vi "Initialize.vi"(8 "error in (no error)":errorcluster, 9 "Reset (True)":bool=TRUE, 10 "ID Query (True)":bool=TRUE, 11 "VISA resource name":refnum<visa-resource-name>) -> (0 "error out":errorcluster, 3 "VISA resource name out":refnum<visa-resource-name>)   [LabVIEW 2010, in "Agilent U2722.lvlib"]
doc: "Establishes communication with the instrument and optionally performs an instrument identification query and/or an instrument reset. It also places the instrument in a default state needed for other instrument driver operations. Therefore, call this VI before calling other instrument driver VIs for this instrument. Generally, you need to call the Initialize VI only once at the beginning of an application."
uses:
  Agilent U2722.lvlib
panel:
  # "(c) 2009 National Instruments.  ALL RIGHTS RESERVED."
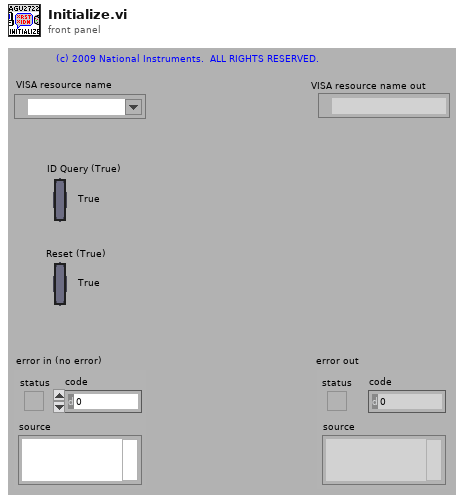
[diagram p1: front panel]
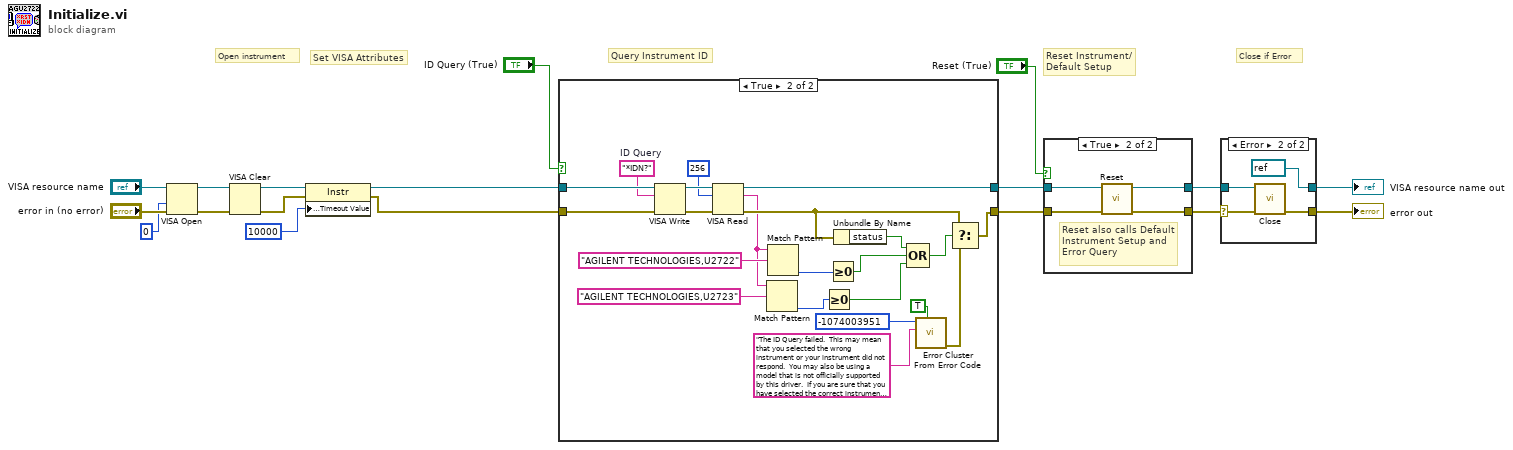
[diagram p0: block diagram]
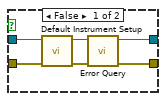
[diagram p3: hidden frame]
diagram:
  # "Set VISA Attributes"
  # "Close if Error"
  # "Query Instrument ID"
  # "Reset Instrument/\nDefault Setup"
  # "Open instrument"
  n1 = VISA Open(access mode=u32 0, error in (no error)="error in (no error)", VISA resource name="VISA resource name") -> (VISA resource name=w10:refnum<visa-resource-name>, error out=w9:errorcluster)  [unwired: 2 in]
  n2 = VISA Clear(VISA resource name=w10, error in (no error)=w9) -> (VISA resource name out=w8:refnum<visa-resource-name>, error out=w7:errorcluster)
  n3 = property class="Instr"(reference=w8, error in=w7, "General Settings:Timeout Value"=u32 10000) -> (reference out=w2:refnum<visa-resource-name>, error out=w1:errorcluster)
  n4 = case shown="True" "ID Query (True)" {
    tunnel: [w19 w42] -> w17
    tunnel: [w20 w39] -> w18
    tunnel: w2 -> [w20 w40]
    tunnel: w1 -> [w19 w41]
    frame False {
    }
    frame True {
      w34 = "*IDN?"  # ID Query
      n5 = VISA Write(VISA resource name=w40, write buffer=w34, error in (no error)=w41) -> (VISA resource name out=w38:refnum<visa-resource-name>, error out=w37:errorcluster)  [unwired: 1 out]
      n6 = VISA Read(VISA resource name=w38, byte count=u32 256, error in (no error)=w37) -> (VISA resource name out=w39:refnum<visa-resource-name>, read buffer=w23:string, error out=w28:errorcluster)  [unwired: 1 out]
      n7 = Match Pattern(string=w23, regular expression="AGILENT TECHNOLOGIES,U2723") -> (offset past match=w22:i32)  [unwired: 1 in, 3 out]
      n8 = Match Pattern(string=w23, regular expression="AGILENT TECHNOLOGIES,U2722") -> (offset past match=w29:i32)  [unwired: 1 in, 3 out]
      n9 = Greater Or Equal To 0?(x=w22) -> (x >= 0?=w21:bool)
      n10 = Greater Or Equal To 0?(x=w29) -> (x >= 0?=w26:bool)
      n11 = Unbundle By Name(w28) -> ("status"=w27:bool)
      n12 = Compound Arithmetic op=OR(w27, w26, w21) -> (w25:bool)
      n13 = call <vilib>:"Error Cluster From Error Code.vi"("show call chain? (False)"=TRUE, "error message (\"\")"="The ID Query failed.  This may mean that you selected the wrong instrument or your instrument did not respond.  You may also be using a model that is not officially supported by this driver.  If you are sure that you have selected the correct instrument and it is responding, try disabling the ID Query." ("Source (VI Name)"), "error code (0)"=-1074003951 ("Code")) -> ("error out"=w33:errorcluster)  [unwired: 6 in]
      n14 = Select(t=w28, s=w25, f=w33) -> (s? t:f=w42:errorcluster)
    }
  }
  n15 = case shown="True" "Reset (True)" {
    tunnel: w17 -> [w47 w49]
    tunnel: [w44 w52] -> w3
    tunnel: w18 -> [w48 w50]
    tunnel: [w45 w51] -> w4
    frame False {
      n16 = call "Default Instrument Setup.vi"("error in (no error)"=w47, "VISA resource name"=w48) -> ("error out"=w43:errorcluster, "VISA resource name out"=w46:refnum<visa-resource-name>)  [unwired: 8 in]
      n17 = call "Error Query.vi"("error in (no error)"=w43, "VISA resource name"=w46) -> ("error out"=w44:errorcluster, "VISA resource name out"=w45:refnum<visa-resource-name>)  [unwired: 6 in, 2 out]
    }
    frame True {
      # "Reset also calls Default Instrument Setup and Error Query"
      n18 = call "Reset.vi"("error in (no error)"=w49, "VISA resource name"=w50) -> ("error out"=w52:errorcluster, "VISA resource name out"=w51:refnum<visa-resource-name>)  [unwired: 8 in]
    }
  }
  n19 = case shown="Error" w3 {
    selector: w3 -> [w53 w56]
    tunnel: w4 -> [w54 w57]
    tunnel: [w54 refnum<visa-resource-name> refnum ("VISA resource name out")] -> w6
    tunnel: [w53 w58] -> w5
    frame No Error {
    }
    frame Error {
      n20 = call "Close.vi"("error in (no error)"=w56, "VISA resource name"=w57) -> ("error out"=w58:errorcluster)  [unwired: 9 in]
    }
  }
  "VISA resource name out" <- w6
  "error out" <- w5
